vi "Clear.vi"(8 "error in (no error)":errorcluster, 11 "Mock Log Handler In":refnum<class "Mock Log Handler.lvclass">) -> (0 "error out":errorcluster)   [LabVIEW 2020, in "Mock Log Handler.lvclass"]
doc: "Clears any resorces allocated during initialization."
uses:
  Mock Log Handler.lvclass
  Mock Log Handler.lvclass/Mock Log Handler.ctl
  Framework/Base/Base.lvclass
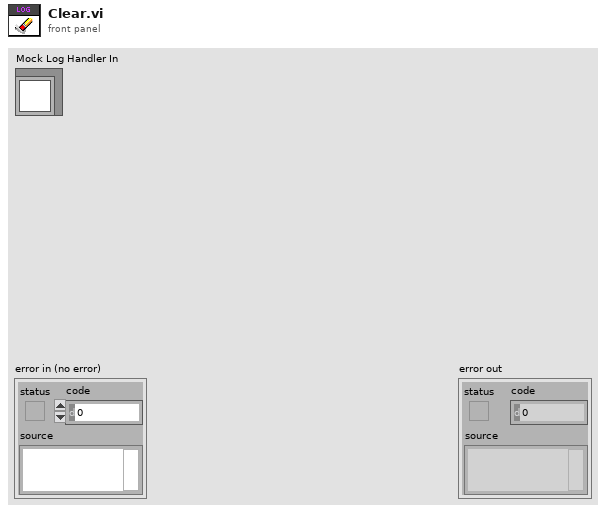
[diagram p1: front panel]
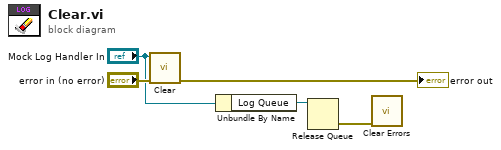
[diagram p0: block diagram]
diagram:
  n1 = call-parent "Clear.vi"("error in (no error)"="error in (no error)", "Base In"="Mock Log Handler In") -> ("error out"=→"error out":errorcluster)  [unwired: 9 in]
  n2 = Unbundle By Name("Mock Log Handler In") -> ("Log Queue"=w3:refnum<queue>)
  n3 = Release Queue(queue=w3) -> (error out=w2:errorcluster)  [unwired: 2 in, 2 out]
  n4 = call <vilib>:"Clear Errors.vi"("error in (no error)"=w2) -> ()  [unwired: 5 in, 2 out]
